vi "Measure - NI 9211.vi"(8 "Error In":errorcluster) -> (0 "Error Out":errorcluster)   [LabVIEW 2011]
uses:
  <vilib>/DAQmx/read.llb/DAQmx Read.vi
  <vilib>/DAQmx/read.llb/DAQmx Read (Analog 1D Wfm NChan NSamp).vi
  <vilib>/DAQmx/miscellaneous.llb/DAQmx Fill In Error Info.vi
panel:
  out "Thermometer":dbl(slide) scale=0.0..100.0
  out "data":waveform(dbl)[](graph) caption="Chart"
  in  "stop":bool
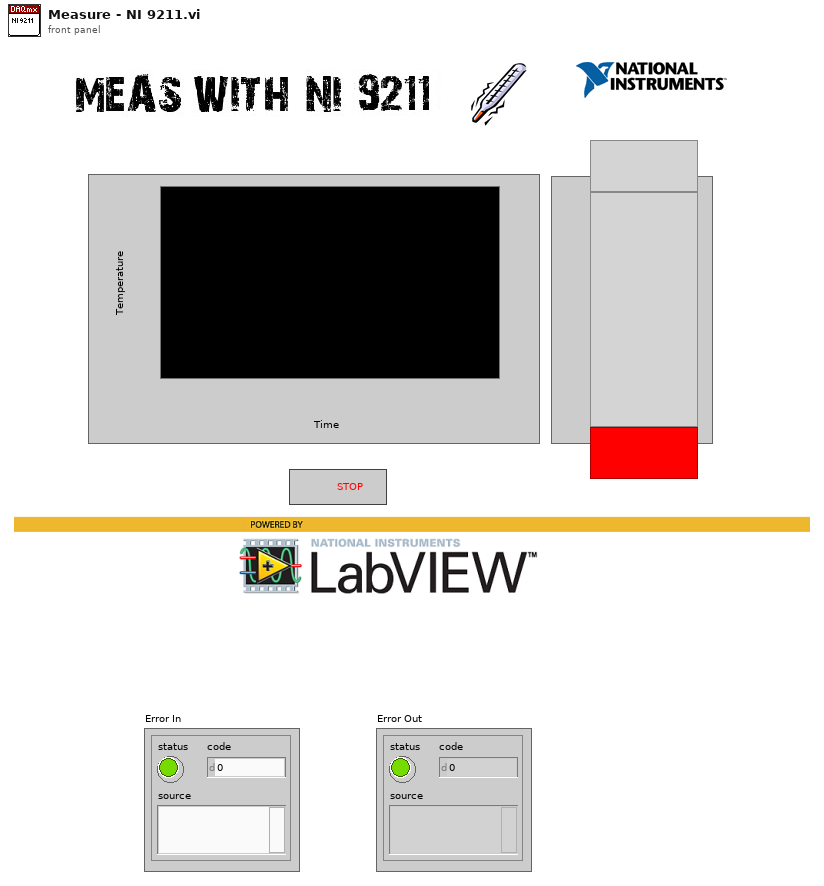
[diagram p1: front panel]
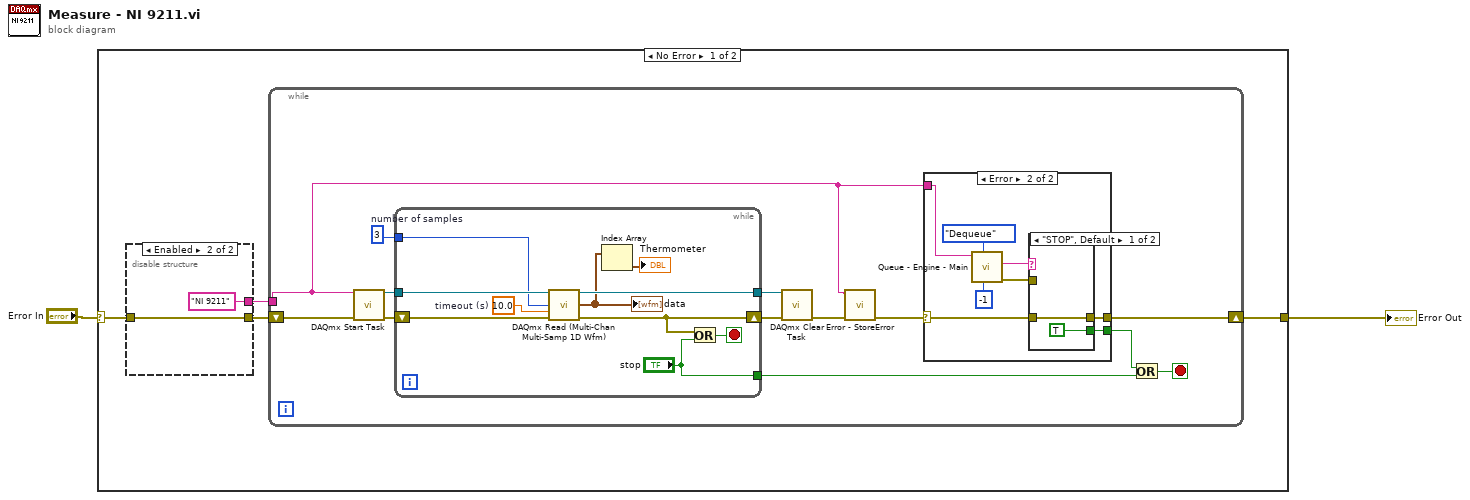
[diagram p0: block diagram]
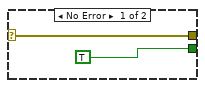
[diagram p2: hidden frame]
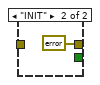
[diagram p3: hidden frame]
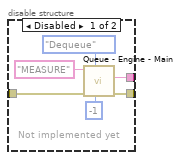
[diagram p4: hidden frame]
diagram:
  n1 = case shown="No Error" "Error In" {
    selector: "Error In" -> [w6 w51]
    tunnel: [w5 w51] -> w2
    frame No Error {
      n2 = disable-structure shown="Enabled" {
        disable-tunnel: [w48 w50] -> w3
        disable-tunnel: [w47 "NI 9211" ("Variable In")] -> w4
        disable-tunnel: w6 -> [w46 w50]
        frame Disabled {
          # "Not implemented yet"
          n3 = call "Queue - Engine - Main.vi"("timeout in ms (-1)"=-1, "Operation"=enum16{"Enqueue", "Dequeue", "Flush", "Release"}."Dequeue", "error in"=w46, "Queue Name In"="MEASURE") -> ("error out"=w48:errorcluster, "Data Out"=w47:string)  [unwired: 5 in, 1 out]
        }
        frame Enabled {
        }
      }
      n4 = while {
        tunnel: w4 -> [w11]
        shift-right: [w10] -> w5
        shift-left: w3 -> [w13]
        stop <- w8 stop-if-true
        w17 = 3  # number of samples
        n5 = call <vilib>:"DAQmx Start Task.vi"("task/channels in"=w11, "error in"=w13) -> ("task out"=w19:refnum<k21>, "error out"=w18:errorcluster)  [unwired: 12 out]
        n6 = while {
          tunnel: w19 -> [w41]
          tunnel: w17 -> [w40]
          tunnel: [w37] -> w15
          shift-right: [w38] -> w16
          shift-left: w18 -> [w39]
          tunnel: ["stop"] -> w7
          stop <- w42 stop-if-true
          w36 = 10.0  # timeout (s)
          n7 = call-poly "DAQmx Read (Multi-Chan Multi-Samp 1D Wfm).vi"("task/channels in"=w41, "number of samples per channel"=w40, "timeout"=w36, "error in"=w39) -> ("task out"=w37:refnum<k21>, "data"=w35:waveform(dbl)[], "error out"=w38:errorcluster)  [unwired: 9 out]
          "data" <- w35
          n8 = Index Array(array=w35) -> (element=→"Thermometer":waveform(dbl))  [unwired: 1 in]
          n9 = Or(x=w38, y="stop") -> (x .or. y?=w42:bool)
        }
        n10 = call <vilib>:"DAQmx Clear Task.vi"("task in"=w15, "error in"=w16) -> ("error out"=w14:errorcluster)  [unwired: 13 out]
        n11 = call "Error - StoreError.vi"("Error In"=w14, "Error Source In"=w11) -> ("Error Out"=w12:errorcluster)  [unwired: 8 in, 1 out]
        n12 = case shown="Error" w12 {
          selector: w12 -> [w21 w22]
          tunnel: [w21 w24] -> w10
          tunnel: [TRUE w23] -> w9
          tunnel: w11 -> [_ w27]
          frame No Error {
          }
          frame Error {
            n13 = call "Queue - Engine - Main.vi"("timeout in ms (-1)"=-1, "Operation"=enum16{"Enqueue", "Dequeue", "Flush", "Release"}."Dequeue", "Queue Name In"=w27) -> ("error out"=w26:errorcluster, "Data Out"=w25:string)  [unwired: 6 in, 1 out]
            n14 = case shown="\"STOP\", Default" w25 {
              tunnel: w26 -> [_ _]
              tunnel: [w30 errorcluster {"status"=FALSE, "code"=0, "source"=""} ("error out")] -> w24
              tunnel: [TRUE _] -> w23
              tunnel: w22 -> [w30 _]
              frame "STOP", Default {
              }
              frame "INIT" {
              }
            }
          }
        }
        n15 = Or(x=w9, y=w7) -> (x .or. y?=w8:bool)
      }
    }
    frame Error {
    }
  }
  "Error Out" <- w2
